vi "Begin.vi"(8 "error in":errorcluster) -> (0 "error out":errorcluster)   [LabVIEW 2018]
doc: "Called before other user functions, this VI is expected to open initial I/O refnums, load in file data, and do all program initialization. Notice that the <B>error out</B> terminal is simply used for data flow. Wiring it to other structures or subVIs ensures that this VI runs first."
uses:
  <vilib>/Rock Robotics/SystemInterfaces/DIO/FPGA_DIOPWMChannel.ctl
  <vilib>/Rock Robotics/WPI/Joystick/WPI_JoystickDeviceEnum.ctl
  <vilib>/Rock Robotics/SystemInterfaces/DIO/FPGA_DIOChannel.ctl
  <vilib>/Rock Robotics/WPI/Solenoid/WPI_SolenoidChannel.ctl
  <vilib>/Rock Robotics/WPI/DriverStation/WPI_DriverStationRobotMode2.ctl
  <vilib>/Rock Robotics/WPI/SafetyOutput/WPI_SafetyOutputConfigMenu.ctl
  <vilib>/Rock Robotics/WPI/Encoder/WPI_EncoderType.ctl
  Robot Global Data.vi
  <vilib>/Rock Robotics/Network Tables/NT Write String Array.vi
  <vilib>/Rock Robotics/WPI/RobotDrive/WPI_RobotDriveOpen4MotorWithSPARK.vi
  <vilib>/Rock Robotics/WPI/MotorControl/WPI_MotorControlOpen VictorSP.vi
  <vilib>/Rock Robotics/WPI/MotorControl/WPI_MotorControlOpen SPARK.vi
  <vilib>/Rock Robotics/WPI/Counter/WPI_CounterDigitalInputToDigitalSource.vi
  <vilib>/Rock Robotics/WPI/Solenoid/WPI_SolenoidOpenDouble.vi
panel:
  in  "JoystickDevice":T1=enum."USB 1"
  in  "B Channel_Stage2":T2=enum."DIO 3"
  in  "A Channel_Stage2":T2=enum."DIO 2"
  in  "B Channel_Stage 1":T2=enum."DIO 5"
  in  "A Channel_Stage1":T2=enum."DIO 4"
  in  "Reverse Solenoid Channel":T3=enum."Solenoid 1"
  in  "Forward Solenoid Channel":T3
  in  "Pneumatics Control Module (0)":u8
  in  "B Channel_Rotation":T2=enum."DIO 1"
  in  "A Channel_Rotation":T2
  in  "Shooter_ArmMotor":T4=enum."PWM 6"
  in  "Rotation_ArmMotor":T4=enum."PWM 7"
  in  "Stage2_Elevator":T4=enum."PWM 4"
  in  "Stage1_Elevator":T4=enum."PWM 5"
  in  "FrontLeft_MotorInverted":bool
  in  "FrontRight_MotorInverted":bool
  in  "RearLeft_MotorInverted":bool
  in  "RearRight_MotorInverted":bool
  in  "Driver Joystick":T1
  in  "FrontRight_DriveMotor":T4=enum."PWM 1"
  in  "FrontLeft_DriveMotor":T4=enum."PWM 2"
  in  "RearRight_DriveMotor":T4
  in  "RearLeft_DriveMotor":T4=enum."PWM 3"
  # "Drive Motors"
  # "Joystick  and Driver Control Reference"
  # "This controller is responsible\nfor controlling the robot\nlift and drive functions"
  # "This controller is responsible\nfor controlling the lift and\nelevator functions when the\nrobot is opperating in \nmanual (manMode)"
  # "Lift/Arm Encoders"
  # "Arm Rotation Encoder"
  # "Set these values to the\nPMW loation on the \nRoboRIO"
  # "When these values are true\nthe signal sent to the drive\nmotors by the motor \ncontroller is inverted. This\nwill keep the motors from\nfighting each other in the\ngearbox"
  # "Arm and Lift Motors"
  # "Arm Pnumatics"
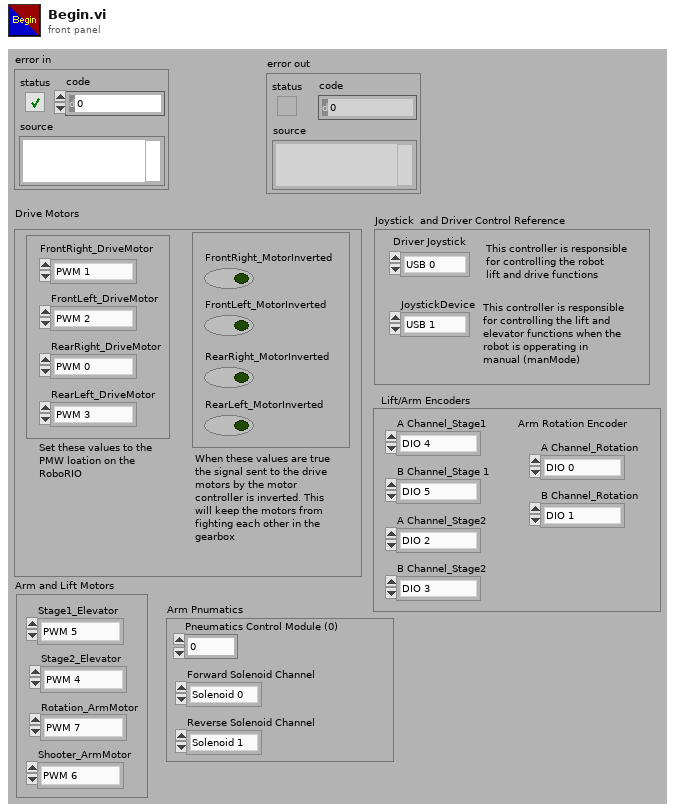
[diagram p1: front panel]
types:
  T1 = typedef "WPI_JoystickDeviceEnum.ctl" = enum16{"USB 0", "USB 1", "USB 2", "USB 3", "USB 4", "USB 5"}
  T2 = typedef "FPGA_DIOChannel.ctl" = enum8{"DIO 0", "DIO 1", "DIO 2", "DIO 3", "DIO 4", "DIO 5", "DIO 6", "DIO 7", "DIO 8", "DIO 9", "DIO MXP 0", "DIO MXP 1", "DIO MXP 2", "DIO MXP 3", "DIO MXP 4", "DIO MXP 5", "DIO MXP 6", "DIO MXP 7", "DIO MXP 8", "DIO MXP 9", "DIO MXP 10", "DIO MXP 11", "DIO MXP 12", "DIO MXP 13", "DIO MXP 14", "DIO MXP 15", "SPI Port CS1", "SPI Port CS2", "SPI Port CS3", "SPI Port MISO", "SPI Port MOSI", "Invalid"}
  T3 = typedef "WPI_SolenoidChannel.ctl" = enum8{"Solenoid 0", "Solenoid 1", "Solenoid 2", "Solenoid 3", "Solenoid 4", "Solenoid 5", "Solenoid 6", "Solenoid 7", "Invalid"}
  T4 = typedef "FPGA_DIOPWMChannel.ctl" = enum8{"PWM 0", "PWM 1", "PWM 2", "PWM 3", "PWM 4", "PWM 5", "PWM 6", "PWM 7", "PWM 8", "PWM 9", "PWM MXP 0", "PWM MXP 1", "PWM MXP 2", "PWM MXP 3", "PWM MXP 4", "PWM MXP 5", "PWM MXP 6", "PWM MXP 7", "PWM MXP 8", "PWM MXP 9", "Invalid"}
  T5 = typedef "WPI_EncoderType.ctl" = enum16{"1x", "2x", "4x"}
  T6 = typedef "WPI_SafetyOutputConfigMenu.ctl" = enum16{"Enable", "Disable"}
  T7 = typedef "WPI_DriverStationRobotMode2.ctl" = enum16{"Autonomous Disabled", "Autonomous Enabled", "Teleop Disabled", "Teleop Enabled", "Disconnected", "Finish", "Test Disabled", "Test Enabled", "Emergency Stopped"}
  T8 = typedef "WPI_MotorControlDeviceRef.ctl" = cluster{"DeviceStatus":errorcluster, "Type":T9, "PWM":cluster{"PWM Channel":T4, "DeadBand":T10}, "CAN":cluster{"Device Number":u8, "SetOutput VI Ref":variant, "GetOutput VI Ref":variant, "Enable VI Ref":variant, "Disable VI Ref":variant, "Data":variant}, "Invert":bool, "DIO PWM":cluster{"PWM \"Enable\" Channel":T4, "DIOChannel":T2, "PWM Rate":dbl}}
  T9 = typedef "WPI_MotorControlType.ctl" = enum16{"PWM", "CAN", "DIO PWM"}
  T10 = typedef "WPI_PWMDeadband.ctl" = cluster{"Name":string, "maxPositivePwm":i32, "minPositivePwm":i32, "centerPwm":i32, "maxNegativePwm":i32, "minNegativePwm":i32, "angularRange":u16}
  T11 = typedef "WPI_JoystickDevRef.ctl" = cluster{"Device":T1}
  T12 = typedef "WPI_SolenoidDevRef.ctl" = cluster{"DevStatus":errorcluster, "Pneumatics Control Module":u8, "Forward Solenoid Channel":T3, "Reverse Solenoid Channel":T3}
  T13 = typedef "WPI_RobotDriveDevRef.ctl" = cluster{"DevStatus":errorcluster, "Motors[]":T8[], "Square Inputs":bool, "Max Output":dbl}
  T14 = typedef "WPI_DigitalInputDevRef.ctl" = cluster{"DevStatus":errorcluster, "DIO Channel":T2}
  T15 = typedef "FPGA_CounterEncoderSourceConvertionLVSourceType.ctl" = cluster{"DevStatus":errorcluster, "AnalogTriggerMode?":bool, "DigitalMode":cluster{"DIO Channel":T16}, "AnalogTriggerMode":cluster{"AnalogTriggerIndex":T17, "OutputType":T18}}
  T16 = typedef "FPGA_DIODigitalSourceChannel.ctl" = enum8{"DIO 0", "DIO 1", "DIO 2", "DIO 3", "DIO 4", "DIO 5", "DIO 6", "DIO 7", "DIO 8", "DIO 9", "DIO MXP 0", "DIO MXP 1", "DIO MXP 2", "DIO MXP 3", "DIO MXP 4", "DIO MXP 5", "DIO MXP 6", "DIO MXP 7", "DIO MXP 8", "DIO MXP 9", "DIO MXP 10", "DIO MXP 11", "DIO MXP 12", "DIO MXP 13", "DIO MXP 14", "DIO MXP 15", "SPI Port CS1", "SPI Port CS2", "SPI Port CS3", "SPI Port MISO", "SPI Port MOSI", "Disabled"}
  T17 = typedef "FPGA_AnalogTriggerIndex.ctl" = enum8{"Trig 0", "Trig 1", "Trig 2", "Trig 3", "Trig 4", "Trig 5", "Trig 6", "Trig 7", "Invalid"}
  T18 = typedef "FPGA_AnalogTriggerOutType.ctl" = enum16{"InWindow", "TriggerState", "Rising", "Falling"}
  T19 = typedef "WPI_EncoderDevRef.ctl" = cluster{"DevStatus":errorcluster, "EncoderIndex":T20, "CounterIndex":T21, "DistancePerCount":dbl, "Decoding Type":T5}
  T20 = typedef "FPGA_EncoderIdx.ctl" = enum8{"Enc 0", "Enc 1", "Enc 2", "Enc 3", "Enc 4", "Enc 5", "Enc 6", "Enc 7", "Invalid"}
  T21 = typedef "FPGA_CounterCtrSystemIndex.ctl" = enum8{"Ctr 0", "Ctr 1", "Ctr 2", "Ctr 3", "Ctr 4", "Ctr 5", "Ctr 6", "Ctr 7", "Invalid"}
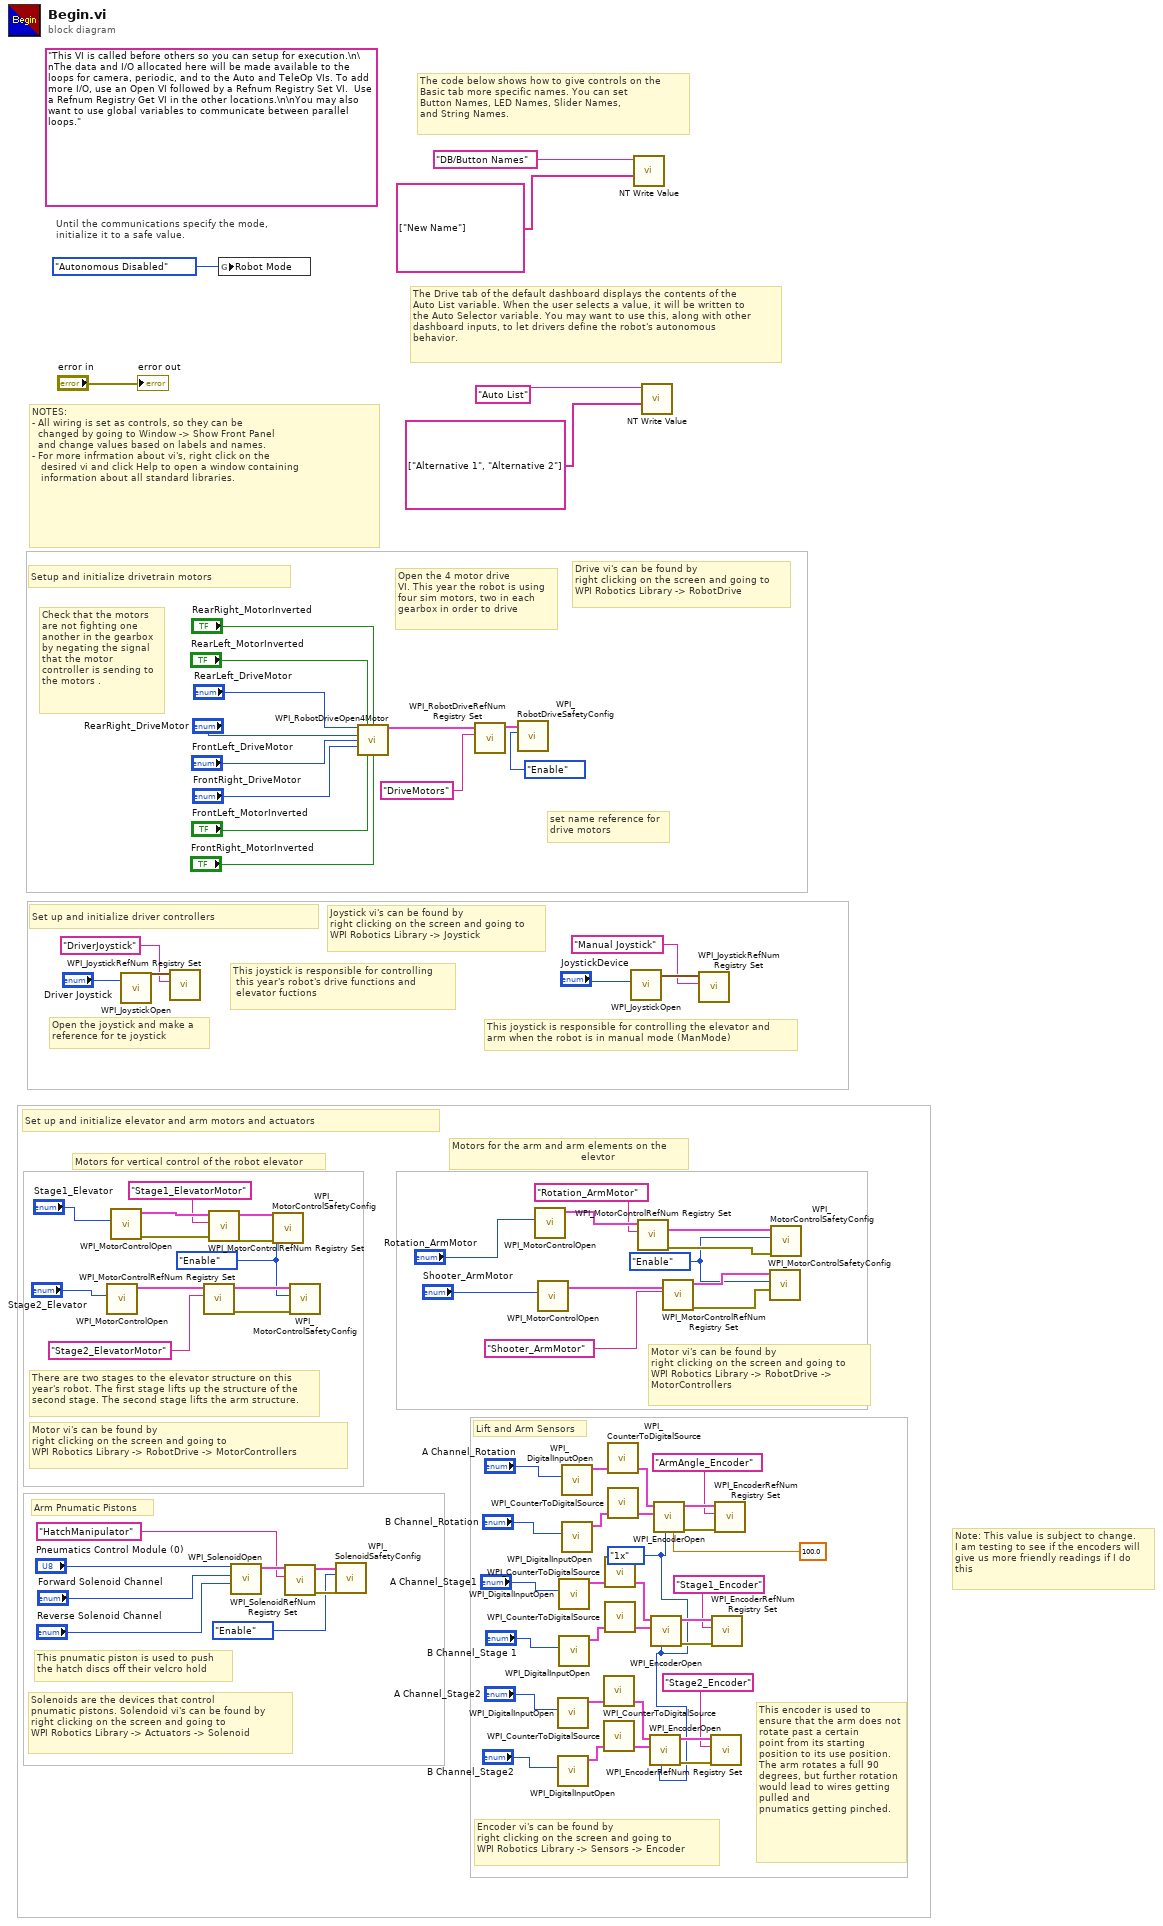
[diagram p0: block diagram]
diagram:
  w10 = WPI_EncoderType."1x" ("Decoding Type")
  w48 = WPI_SafetyOutputConfigMenu."Enable" ("mode")
  w58 = WPI_SafetyOutputConfigMenu."Enable" ("mode")
  (unwired) "This VI is called before others so you can setup for execution.\n\nThe data and I/O allocated here will be made available to the loops for camera, periodic, and to the Auto and TeleOp VIs. To add more I/O, use an Open VI followed by a Refnum Registry Set VI.  Use a Refnum Registry Get VI in the other locations.\n\nYou may also want to use global variables to communicate between parallel loops."
  # "This joystick is responsible for controlling the elevator and \narm when the robot is in manual mode (ManMode)"
  # "Note: This value is subject to change.\nI am testing to see if the encoders will\ngive us more friendly readings if I do\nthis"
  # "Encoder vi's can be found by\nright clicking on the screen and going to \nWPI Robotics Library -> Sensors -> Encoder"
  # "Solenoids are the devices that control\npnumatic pistons. Solendoid vi's can be found by\nright clicking on the screen and going to\nWPI Robotics Library -> Actuators -> Solenoid"
  # "Motor vi's can be found by\nright clicking on the screen and going to\nWPI Robotics Library -> RobotDrive -> \nMotorControllers"
  # "Motor vi's can be found by\nright clicking on the screen and going to\nWPI Robotics Library -> RobotDrive -> MotorControllers"
  # "Joystick vi's can be found by \nright clicking on the screen and going to\nWPI Robotics Library -> Joystick"
  # "Drive vi's can be found by \nright clicking on the screen and going to\nWPI Robotics Library -> RobotDrive"
  # "Open the joystick and make a\nreference for te joystick"
  # "NOTES:\n- All wiring is set as controls, so they can be\n  changed by going to Window -> Show Front Panel\n  and change values based on labels and names.\n- For more infrmation about vi's, right click on the \n   desired vi and click Help to open a window containing\n   information about all standard libraries."
  # "This pnumatic piston is used to push\nthe hatch discs off their velcro hold"
  # "Arm Pnumatic Pistons"
  # "This encoder is used to ensure that the arm does not rotate past a certain\npoint from its starting position to its use position. The arm rotates a full 90 degrees, but further rotation would lead to wires getting pulled and \npnumatics getting pinched."
  # "Lift and Arm Sensors"
  # "There are two stages to the elevator structure on this\nyear's robot. The first stage lifts up the structure of the\nsecond stage. The second stage lifts the arm structure."
  # "Motors for the arm and arm elements on the\n                                           elevtor"
  # "Motors for vertical control of the robot elevator"
  # "Set up and initialize elevator and arm motors and actuators"
  # "This joystick is responsible for controlling\n this year's robot's drive functions and\n elevator fuctions"
  # "Set up and initialize driver controllers"
  # "Check that the motors\nare not fighting one \nanother in the gearbox\nby negating the signal \nthat the motor \ncontroller is sending to\nthe motors ."
  # "Open the 4 motor drive\nVI. This year the robot is using\nfour sim motors, two in each\ngearbox in order to drive"
  # "set name reference for\ndrive motors"
  # "Setup and initialize drivetrain motors"
  # "The Drive tab of the default dashboard displays the contents of the\nAuto List variable. When the user selects a value, it will be written to\nthe Auto Selector variable. You may want to use this, along with other\ndashboard inputs, to let drivers define the robot's autonomous\nbehavior."
  # "The code below shows how to give controls on the\nBasic tab more specific names. You can set\nButton Names, LED Names, Slider Names,\nand String Names."
  # "Until the communications specify the mode,\ninitialize it to a safe value."
  n1 = call-poly <vilib>:"WPI_MotorControlOpen.vi"("PWM Channel"="Stage2_Elevator") -> ("MotorControlDeviceRef"=w64:T8)  [unwired: 9 in, 1 out]
  n2 = call-poly <vilib>:"WPI_MotorControlOpen.vi"("PWM Channel"="Stage1_Elevator") -> ("error out"=w62:errorcluster, "MotorControlDeviceRef"=w65:T8)  [unwired: 9 in]
  n3 = call <vilib>:"WPI_JoystickOpen.vi"("JoystickDevice"="Driver Joystick") -> ("JoystickDevRef"=w71:T11)  [unwired: 10 in]
  n4 = call <vilib>:"WPI_JoystickRefNum Registry Set.vi"("refnum name"="DriverJoystick", "JoystickDevRef"=w71) -> ()  [unwired: 8 in, 2 out]
  n5 = call <vilib>:"WPI_MotorControlRefNum Registry Set.vi"("refnum name"="Stage2_ElevatorMotor", "MotorControlDevRef"=w64) -> ("error out"=w59:errorcluster, "MotorControlDevRef"=w60:T8)  [unwired: 8 in]
  n6 = call <vilib>:"WPI_MotorControlRefNum Registry Set.vi"("error in (no error)"=w62, "refnum name"="Stage1_ElevatorMotor", "MotorControlDevRef"=w65) -> ("error out"=w61:errorcluster, "MotorControlDevRef"=w6:T8)  [unwired: 7 in]
  n7 = global write "Robot Global Data.vi" "Robot Mode"(WPI_DriverStationRobotMode2."Autonomous Disabled" ("Robot Mode")) -> ()
  n8 = call-poly <vilib>:"WPI_SolenoidOpen.vi"("Reverse Solenoid Channel"="Reverse Solenoid Channel", "Forward Solenoid Channel"="Forward Solenoid Channel", "Pneumatics Control Module (0)"="Pneumatics Control Module (0)") -> ("SolenoidDevRef"=w38:T12)  [unwired: 7 in, 1 out]
  n9 = call <vilib>:"WPI_MotorControlSafetyConfig.vi"("error in (no error)"=w61, "mode"=w58, "MotorControlDevRef"=w6) -> ()  [unwired: 7 in, 2 out]
  n10 = call <vilib>:"WPI_SolenoidRefNum Registry Set.vi"("refnum name"="HatchManipulator", "SolenoidDevRef"=w38) -> ("error out"=w36:errorcluster, "SolenoidDevRef"=w35:T12)  [unwired: 8 in]
  n11 = call <vilib>:"WPI_MotorControlSafetyConfig.vi"("error in (no error)"=w59, "mode"=w58, "MotorControlDevRef"=w60) -> ()  [unwired: 7 in, 2 out]
  n12 = call <vilib>:"WPI_SolenoidSafetyConfig.vi"("error in (no error)"=w36, "mode"=WPI_SafetyOutputConfigMenu."Enable", "SolenoidDevRef"=w35) -> ()  [unwired: 7 in, 2 out]
  n13 = call-poly <vilib>:"WPI_RobotDriveOpen4Motor.vi"("Rear Left Motor"="RearLeft_DriveMotor", "Rear Left Motor Inverted"="RearLeft_MotorInverted", "Rear Right Motor Inverted"="RearRight_MotorInverted", "Rear Right Motor"="RearRight_DriveMotor", "Front Left Motor"="FrontLeft_DriveMotor", "Front Right Motor"="FrontRight_DriveMotor", "Front Left Motor Inverted"="FrontLeft_MotorInverted", "Front Right Motor Inverted"="FrontRight_MotorInverted") -> ("RobotDriveDevRef"=w78:T13)  [unwired: 6 in, 1 out]
  n14 = call <vilib>:"WPI_RobotDriveRefNum Registry Set.vi"("refnum name"="DriveMotors", "RobotDriveDevRef"=w78) -> ("RobotDriveDevRef"=w77:T13)  [unwired: 8 in, 1 out]
  n15 = call <vilib>:"WPI_RobotDriveSafetyConfig.vi"("mode"=WPI_SafetyOutputConfigMenu."Enable", "RobotDriveDevRef"=w77) -> ()  [unwired: 8 in, 2 out]
  n16 = call-poly <vilib>:"WPI_MotorControlOpen.vi"("PWM Channel"="Rotation_ArmMotor") -> ("MotorControlDeviceRef"=w57:T8)  [unwired: 9 in, 1 out]
  n17 = call-poly <vilib>:"WPI_MotorControlOpen.vi"("PWM Channel"="Shooter_ArmMotor") -> ("MotorControlDeviceRef"=w52:T8)  [unwired: 9 in, 1 out]
  n18 = call <vilib>:"WPI_DigitalInputOpen.vi"("DIO Channel"="A Channel_Stage2") -> ("DigitalInputDevRef"=w27:T14)  [unwired: 1 in, 9 out]
  n19 = call <vilib>:"WPI_DigitalInputOpen.vi"("DIO Channel"="B Channel_Stage2") -> ("DigitalInputDevRef"=w28:T14)  [unwired: 1 in, 9 out]
  n20 = call <vilib>:"WPI_DigitalInputOpen.vi"("DIO Channel"="A Channel_Stage1") -> ("DigitalInputDevRef"=w15:T14)  [unwired: 1 in, 9 out]
  n21 = call <vilib>:"WPI_DigitalInputOpen.vi"("DIO Channel"="B Channel_Stage 1") -> ("DigitalInputDevRef"=w16:T14)  [unwired: 1 in, 9 out]
  n22 = call <vilib>:"WPI_DigitalInputOpen.vi"("DIO Channel"="A Channel_Rotation") -> ("DigitalInputDevRef"=w43:T14)  [unwired: 1 in, 9 out]
  n23 = call <vilib>:"WPI_DigitalInputOpen.vi"("DIO Channel"="B Channel_Rotation") -> ("DigitalInputDevRef"=w44:T14)  [unwired: 1 in, 9 out]
  n24 = call-poly <vilib>:"WPI_CounterToDigitalSource.vi"("DigitalInputDevRef"=w27) -> ("Digital Source"=w26:T15)  [unwired: 6 out]
  n25 = call-poly <vilib>:"WPI_CounterToDigitalSource.vi"("DigitalInputDevRef"=w28) -> ("Digital Source"=w29:T15)  [unwired: 6 out]
  n26 = call-poly <vilib>:"WPI_CounterToDigitalSource.vi"("DigitalInputDevRef"=w15) -> ("Digital Source"=w14:T15)  [unwired: 6 out]
  n27 = call-poly <vilib>:"WPI_CounterToDigitalSource.vi"("DigitalInputDevRef"=w16) -> ("Digital Source"=w17:T15)  [unwired: 6 out]
  n28 = call-poly <vilib>:"WPI_CounterToDigitalSource.vi"("DigitalInputDevRef"=w43) -> ("Digital Source"=w42:T15)  [unwired: 6 out]
  n29 = call-poly <vilib>:"WPI_CounterToDigitalSource.vi"("DigitalInputDevRef"=w44) -> ("Digital Source"=w45:T15)  [unwired: 6 out]
  n30 = call <vilib>:"WPI_JoystickOpen.vi"("JoystickDevice"="JoystickDevice") -> ("JoystickDevRef"=w22:T11)  [unwired: 10 in]
  n31 = call-poly <vilib>:"NT Write Value.vi"("String Array"=string[] ["New Name"], "Name"="DB/Button Names") -> ()  [unwired: 9 in, 1 out]
  n32 = call <vilib>:"WPI_MotorControlRefNum Registry Set.vi"("refnum name"="Rotation_ArmMotor", "MotorControlDevRef"=w57) -> ("error out"=w53:errorcluster, "MotorControlDevRef"=w54:T8)  [unwired: 8 in]
  n33 = call-poly <vilib>:"NT Write Value.vi"("String Array"=string[] ["Alternative 1", "Alternative 2"], "Name"="Auto List") -> ()  [unwired: 9 in, 1 out]
  n34 = call <vilib>:"WPI_EncoderOpen.vi"("Decoding Type"=w10, "BSource"=w29, "ASource"=w26) -> ("error out"=w25:errorcluster, "EncoderDevRef"=w24:T19)  [unwired: 5 in, 2 out]
  n35 = call <vilib>:"WPI_EncoderOpen.vi"("Decoding Type"=w10, "BSource"=w17, "ASource"=w14) -> ("error out"=w13:errorcluster, "EncoderDevRef"=w12:T19)  [unwired: 5 in, 2 out]
  n36 = call <vilib>:"WPI_EncoderOpen.vi"("DistancePerCount"=100.0, "Decoding Type"=w10, "BSource"=w45, "ASource"=w42) -> ("error out"=w41:errorcluster, "EncoderDevRef"=w40:T19)  [unwired: 4 in, 2 out]
  n37 = call <vilib>:"WPI_MotorControlRefNum Registry Set.vi"("refnum name"="Shooter_ArmMotor", "MotorControlDevRef"=w52) -> ("error out"=w3:errorcluster, "MotorControlDevRef"=w49:T8)  [unwired: 8 in]
  n38 = call <vilib>:"WPI_JoystickRefNum Registry Set.vi"("refnum name"="Manual Joystick", "JoystickDevRef"=w22) -> ()  [unwired: 8 in, 2 out]
  n39 = call <vilib>:"WPI_EncoderRefNum Registry Set.vi"("error in (no error)"=w25, "refnum name"="Stage2_Encoder", "EncoderDevRef"=w24) -> ()  [unwired: 7 in, 2 out]
  n40 = call <vilib>:"WPI_EncoderRefNum Registry Set.vi"("error in (no error)"=w13, "refnum name"="Stage1_Encoder", "EncoderDevRef"=w12) -> ()  [unwired: 7 in, 2 out]
  n41 = call <vilib>:"WPI_EncoderRefNum Registry Set.vi"("error in (no error)"=w41, "refnum name"="ArmAngle_Encoder", "EncoderDevRef"=w40) -> ()  [unwired: 7 in, 2 out]
  n42 = call <vilib>:"WPI_MotorControlSafetyConfig.vi"("error in (no error)"=w3, "mode"=w48, "MotorControlDevRef"=w49) -> ()  [unwired: 7 in, 2 out]
  n43 = call <vilib>:"WPI_MotorControlSafetyConfig.vi"("error in (no error)"=w53, "mode"=w48, "MotorControlDevRef"=w54) -> ()  [unwired: 7 in, 2 out]
  "error out" <- "error in"
